vi "Read Payload.vi"(8 "error in (no error)":errorcluster, 11 "CIF_NIChn_Fifo_U8 in":refnum<class "CIF_NIChn_Fifo_U8.lvclass">) -> (0 "error out":errorcluster, 2 "Payload":u8[](array[numeric]) format="%.0x", 3 "CIF_NIChn_Fifo_U8 out":refnum<class "CIF_NIChn_Fifo_U8.lvclass">)   [LabVIEW 2021, in "CIF_NIChn_Fifo_U8.lvclass"]
uses:
  CIF_NIChn_Fifo_U8.lvclass
  CIF_NIChn_Fifo_U8.lvclass/CIF_NIChn_Fifo_U8.ctl
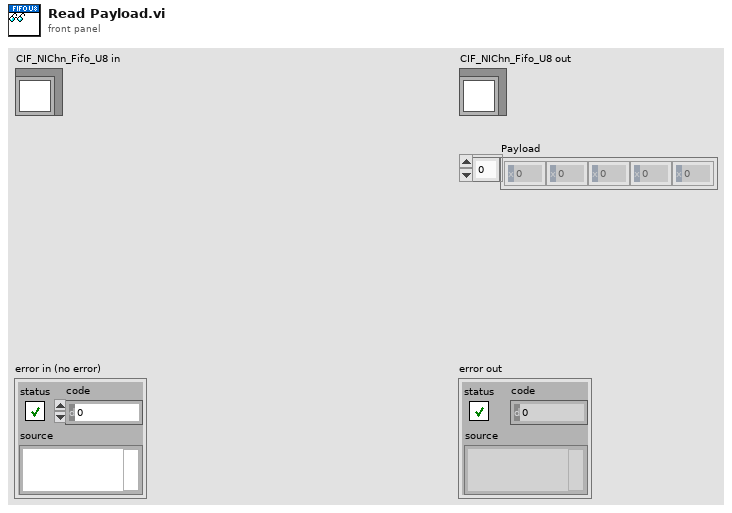
[diagram p1: front panel]
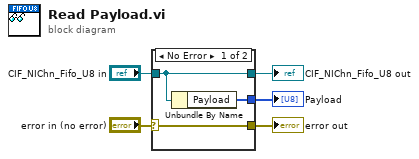
[diagram p0: block diagram]
diagram:
  n1 = case shown="No Error" "error in (no error)" {
    selector: "error in (no error)" -> [w8 w9]
    tunnel: [w8 w9] -> w4
    tunnel: [w7 w10] -> w2
    tunnel: "CIF_NIChn_Fifo_U8 in" -> [w7 w10]
    tunnel: [w6 _] -> w1
    frame No Error {
      n2 = Unbundle By Name(w7) -> ("Payload"=w6:u8[])
    }
    frame Error {
    }
  }
  "error out" <- w4
  "CIF_NIChn_Fifo_U8 out" <- w2
  "Payload" <- w1
